vi "SMART_GenericProcess.vi"() -> ()   [LabVIEW 2017]
uses:
  <vilib>/Utility/miscctls.llb/LVPointTypeDef.ctl
panel:
  in  "Bool数据源":bool
  out "数据源预览":string
  in  "Smart预处理":string[][](array[string])
  in  "数据源什么类型？":enum16{"String类型", "NUM类型", "Bool类型"}(ring)
  in  "String数据源":string
  out "预处理后文本":string
  in  "Smart发送预处理btn":bool
  in  "NUM数据源":dbl
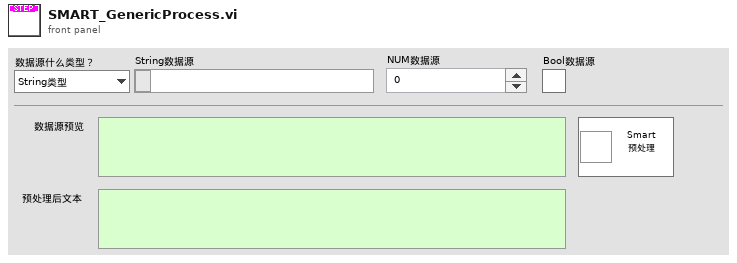
[diagram p1: front panel]
types:
  T1 = typedef "LVPointTypeDef.ctl" = cluster{"Horizontal":i16, "Vertical":i16}
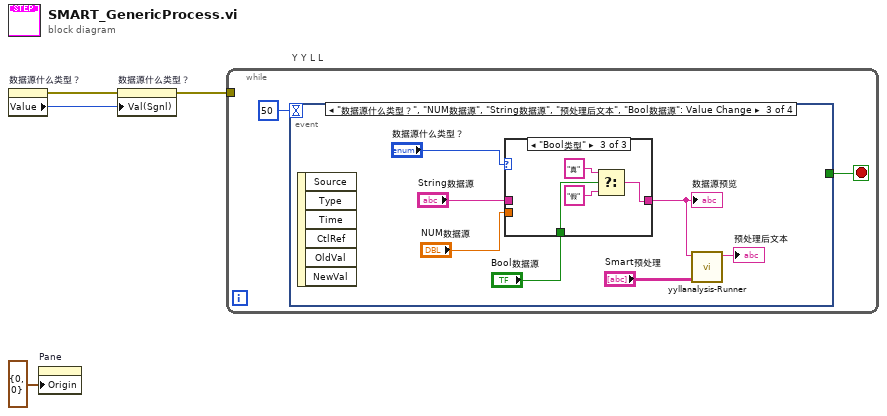
[diagram p0: block diagram]
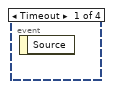
[diagram p2: hidden frame]
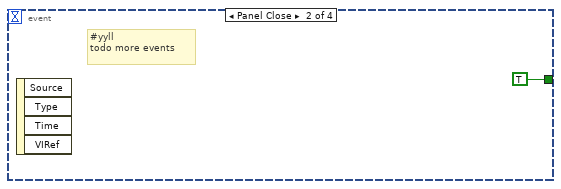
[diagram p3: hidden frame]
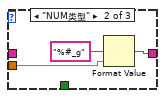
[diagram p5: hidden frame]
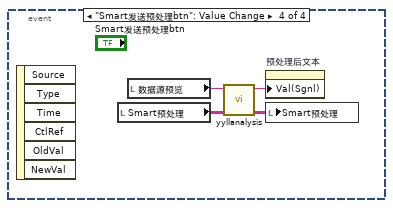
[diagram p6: hidden frame]
diagram:
  # "Y Y L L"
  n1 = property on="数据源什么类型？" class="Enum (strict)"() -> (error out=w1:errorcluster, "Value"=w3:enum16{"String类型", "NUM类型", "Bool类型"})  [unwired: 2 in, 1 out]
  n2 = property on="Pane" class="Pane"("Origin"=T1 {"Horizontal"=0, "Vertical"=0}) -> ()  [unwired: 2 in, 2 out]
  n3 = property on="数据源什么类型？" class="Enum (strict)"(error in=w1, "Val(Sgnl)"=w3) -> (error out=w2:errorcluster)  [unwired: 1 in, 1 out]
  n4 = while {
    tunnel: w2 -> [_]
    stop <- w5 stop-if-true
    n5 = event shown="[2] \"数据源什么类型？\", \"NUM数据源\", \"String数据源\", \"预处理后文本\", \"Bool数据源\": Value Change" {
      selector: _ -> [_ _ _ _]
      dyn-events: _ -> [_ _ _ _]
      timeout: 50 -> [_ _ _ _]
      tunnel: [_ TRUE ("Discard?") _ _] -> w5
      event Timeout {
        n6 = event-data() -> ()  [unwired: 1 in, 1 out]
      }
      event Panel Close {
        # "#yyll\ntodo more events"
        n7 = event-data() -> ()  [unwired: 1 in, 4 out]
      }
      event "数据源什么类型？", "NUM数据源", "String数据源", "预处理后文本", "Bool数据源": Value Change {
        n8 = event-data() -> ()  [unwired: 1 in, 6 out]
        n9 = case shown="\"Bool类型\"" "数据源什么类型？" {
          tunnel: "String数据源" -> [w15 _ _]
          tunnel: [w15 w17 w20] -> w9
          tunnel: "NUM数据源" -> [_ w18 _]
          tunnel: "Bool数据源" -> [_ _ w19]
          frame "String类型" {
          }
          frame "NUM类型" {
            n10 = Format Value(format string="%#_g", value (0)=w18) -> (output string=w17:string)  [unwired: 1 in]
          }
          frame "Bool类型" {
            n11 = Select(t="真", s=w19, f="假") -> (s? t:f=w20:string)
          }
        }
        "数据源预览" <- w9
        n12 = call "yyllanalysis-Runner.vi"("inputs"="Smart预处理", "String in"=w9) -> ("String out"=→"预处理后文本":string)  [unwired: 8 in, 1 out]
      }
      event "Smart发送预处理btn": Value Change {
        n13 = event-data() -> ()  [unwired: 1 in, 6 out]
        n14 = local read "Smart预处理"() -> (w26:string[][])
        n15 = local read "数据源预览"() -> (w24:string)
        n16 = call "yyllanalysis.vi"("Datain"=w26, "StringIN"=w24) -> ("Dataout"=w25:string[][], "StringOUT"=w23:string)  [unwired: 8 in]
        n17 = property on="预处理后文本" class="Str"("Val(Sgnl)"=w23) -> ()  [unwired: 2 in, 2 out]
        n18 = local write "Smart预处理"(w25) -> ()
      }
    }
  }
